vi "Release VIs From Memory.vi"(0 "Current open project IN":refnum<vi>, 11 "error in (no error)":errorcluster) -> (4 "Current open project OUT":refnum<vi>, 15 "error out":errorcluster)   [LabVIEW 2019, in "SolutionBuilder.lvlib"]
uses:
  SolutionBuilder/SolutionBuilder.lvlib
  <vilib>/Utility/EditLVProj/Edit LVProj.lvlib
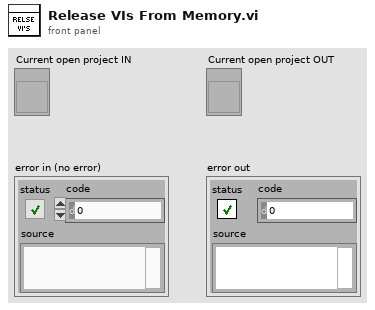
[diagram p1: front panel]
types:
  T1 = typedef "Edit LVProj.lvlib/Library And VI References.ctl" = cluster{"Target Reference":refnum<vi>, "VI References":refnum<vi>[], "Library References":refnum<vi>[]}
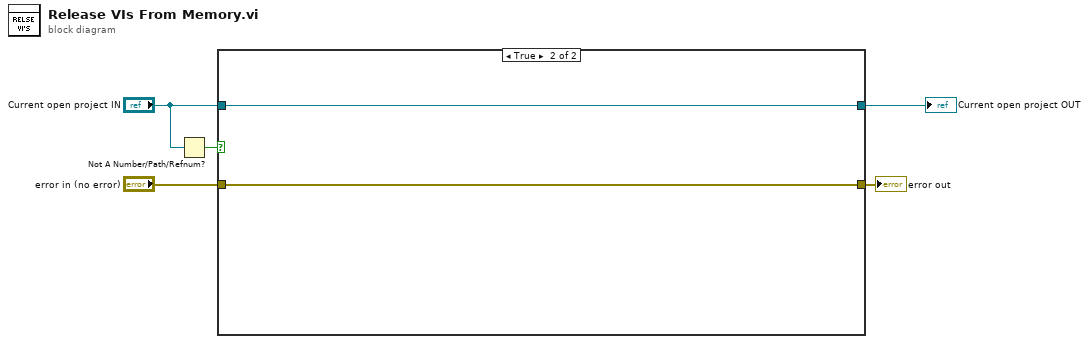
[diagram p0: block diagram]
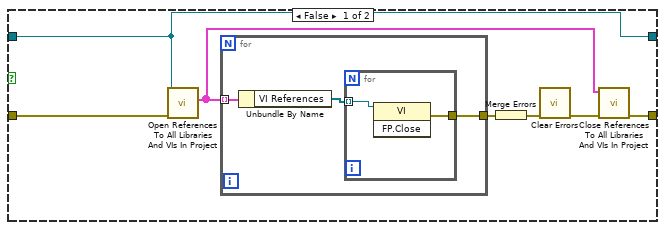
[diagram p2: hidden frame]
diagram:
  n1 = Not A Number/Path/Refnum?(number/path/refnum="Current open project IN") -> (NaN/Path/Refnum?=w1:bool)
  n2 = case shown="True" w1 {
    tunnel: [w8 w18] -> w5
    tunnel: "Current open project IN" -> [w7 w19]
    tunnel: [w7 w19] -> w4
    tunnel: "error in (no error)" -> [w6 w18]
    frame False {
      n3 = call <vilib>:"Open References To All Libraries And VIs In Project.vi"("error in (no error)"=w6, "Project in"=w7) -> ("VI and Library References"=w12:T1[])  [unwired: 7 in, 2 out]
      n4 = for {
        tunnel: w12 -> [w15] mode=indexing
        tunnel: [w13] -> w11
        n5 = Unbundle By Name(w15) -> ("VI References"=w14:refnum<vi>[])
        n6 = for {
          tunnel: w14 -> [w17] mode=indexing
          tunnel: [w16] -> w13
          n7 = invoke class="VI" method="FP.Close"(reference=w17) -> (error out=w16:errorcluster)  [unwired: 2 in, 2 out]
        }
      }
      n8 = Merge Errors(w11) -> (w10:errorcluster)
      n9 = call <vilib>:"Clear Errors.vi"("error in (no error)"=w10) -> ("error out"=w9:errorcluster)  [unwired: 5 in, 1 out]
      n10 = call <vilib>:"Close References To All Libraries And VIs In Project.vi"("error in (no error)"=w9, "VI and Library References"=w12) -> ("error out"=w8:errorcluster)  [unwired: 9 in]
    }
    frame True {
    }
  }
  "error out" <- w5
  "Current open project OUT" <- w4
